vi "QAQC_vacoff.vi"() -> ()   [LabVIEW 2015]
uses:
  GlobalPath.vi
  GlobalData.vi
  GlobalVi.vi
panel:
  out "Mapping file Int sx":string
  out "Mapping file Int dx":string
  out "Mapping file Ext sx":string
  out "Mapping file Ext dx":string
  out "Mapping file pillar":string
  out "PanelName":string
  in  "DONE ALL?":bool
  in  "ptfe 6":bool caption="Open the vi for the QAQC planarity measurements of the frame+cooling bar region"
  in  "ptfe 3":bool caption="Remove the tooling from the table"
  in  "ptfe 5":bool caption="Open the vi for the QAQC planarity measurements of the pillar region"
  in  "ptfe 2":bool caption="Make sure the vacuum is switched OFF"
  # "1. QAQC with vacuum off"
  # "2. Start QAQC process"
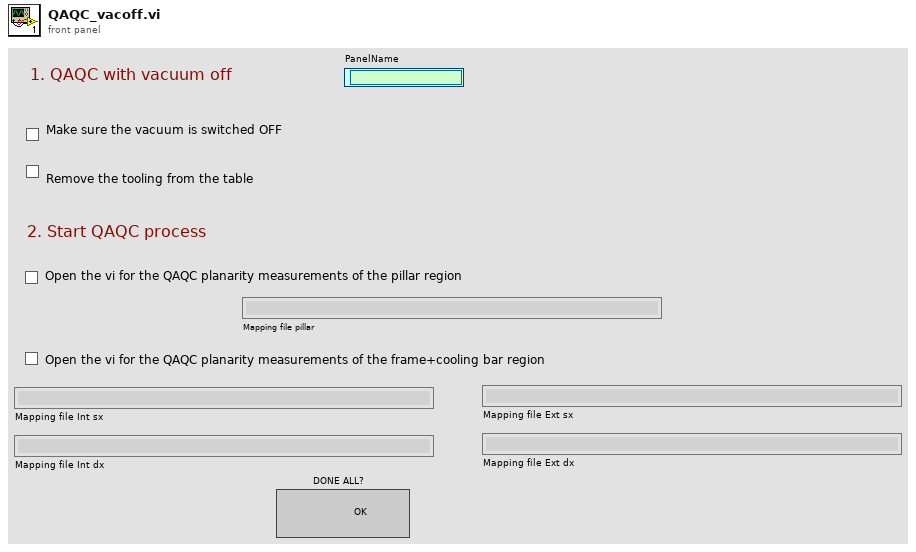
[diagram p1: front panel]
types:
  T1 = enum16{"open", "replace", "create", "open or create", "replace or create", "replace or create with confirmation"}
  T2 = enum32{"Bad", "Idle", "Run top level", "Running"}
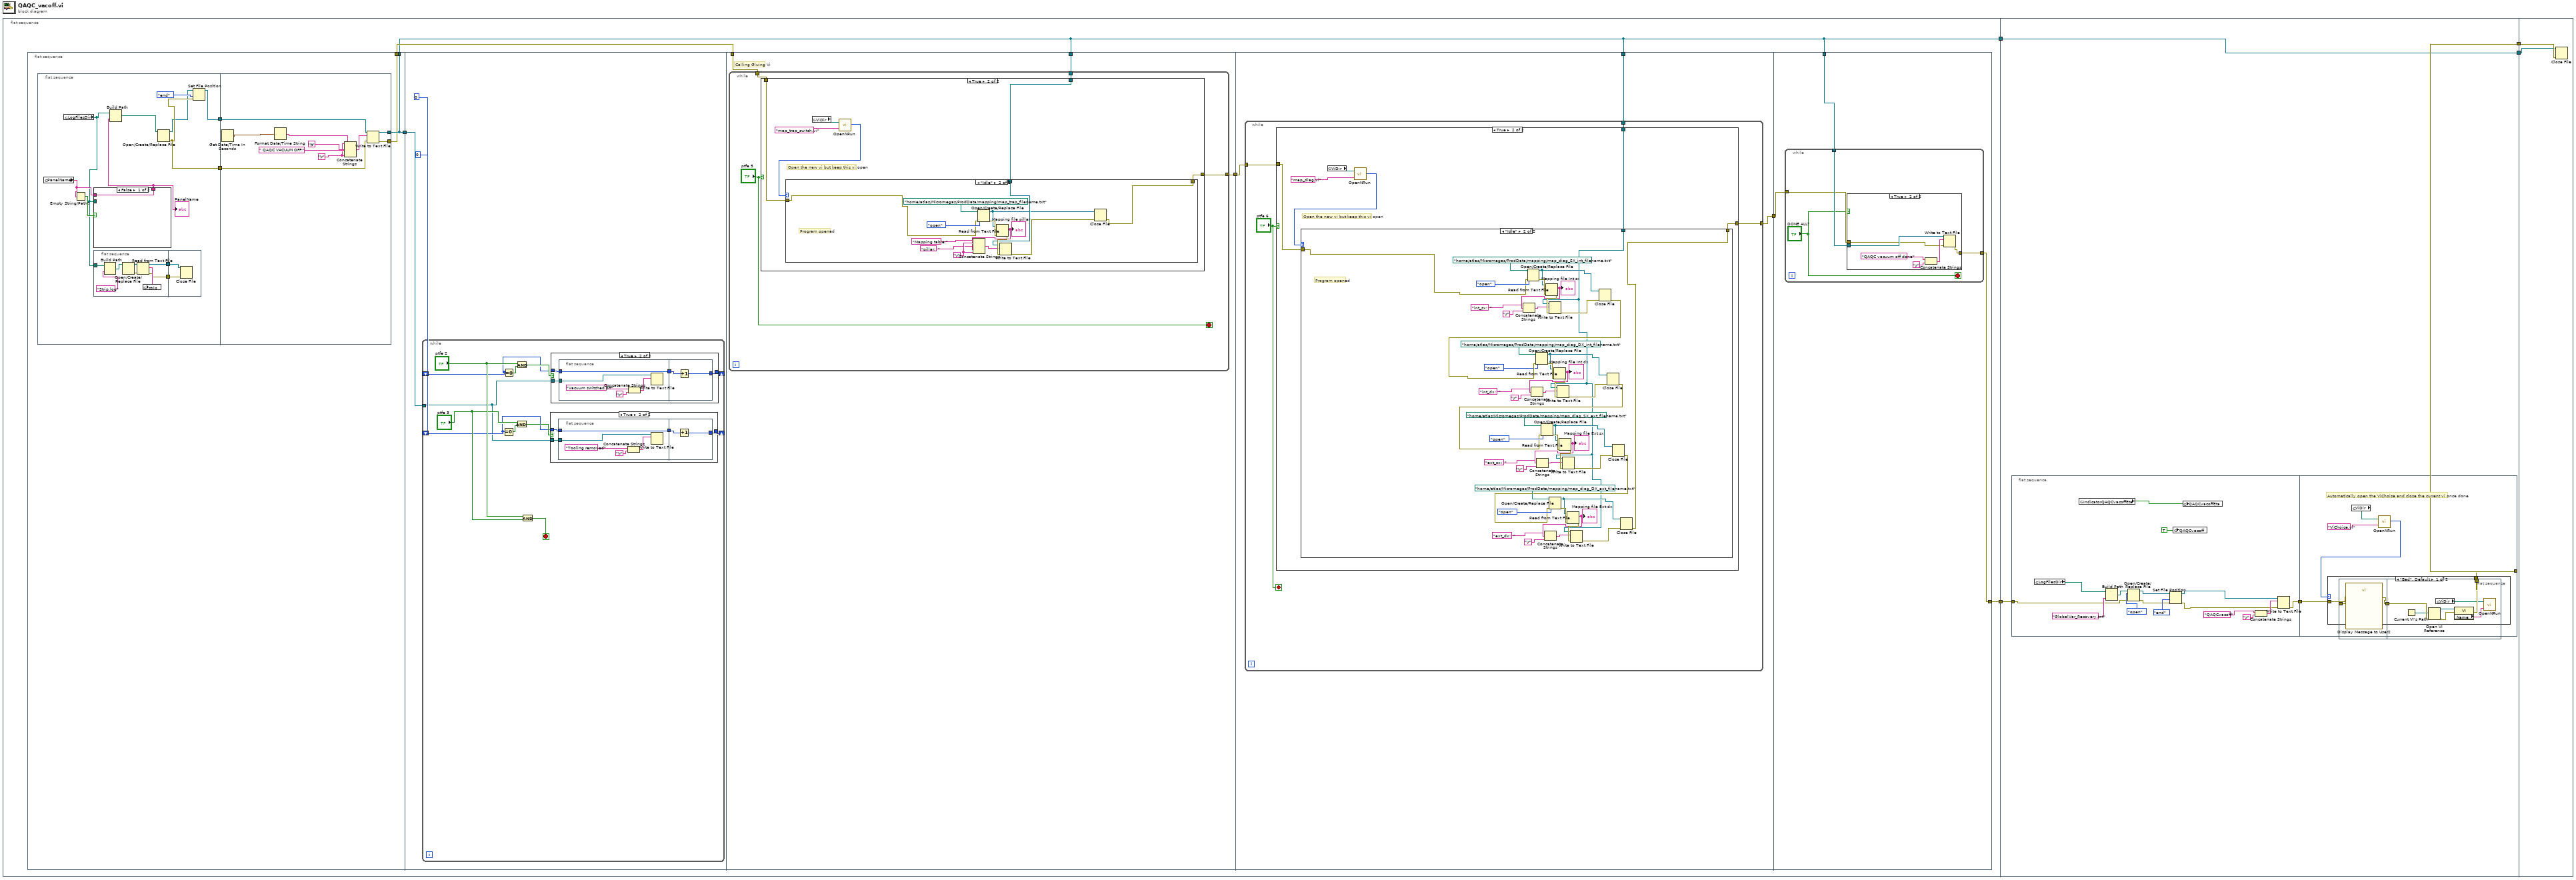
[diagram p0: block diagram]
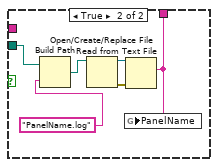
[diagram p2: hidden frame]
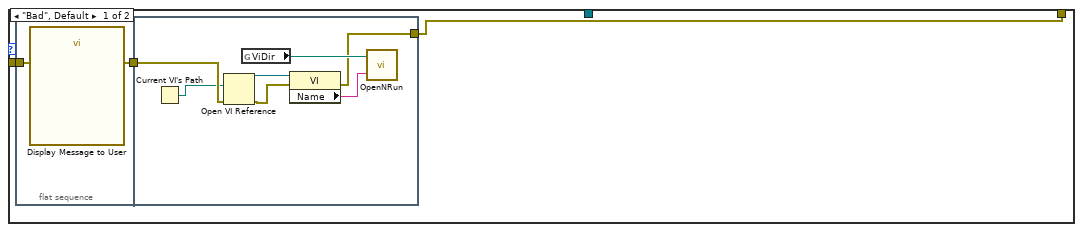
[diagram p6: hidden frame]
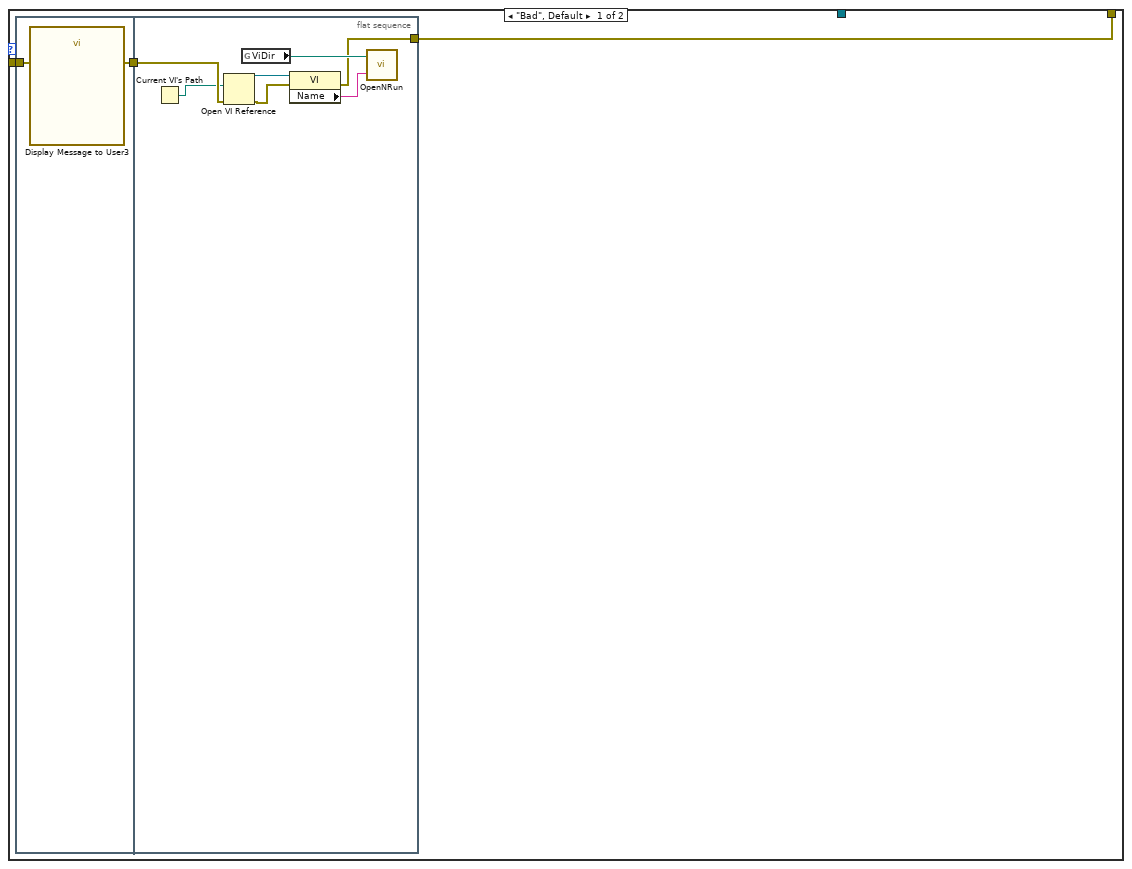
[diagram p8: hidden frame]
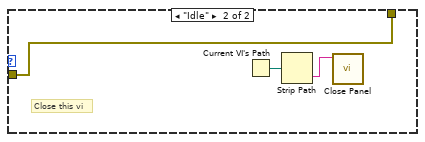
[diagram p10: hidden frame]
diagram:
  n1 = flat-sequence {
    tunnel: [w5] -> w3
    tunnel: [w6] -> w1
    tunnel: [w221] -> w4
    tunnel: w3 -> [w220]
    tunnel: [w220] -> w2
    tunnel: w1 -> [w218]
    tunnel: w4 -> [w259]
    tunnel: w2 -> [w258]
    frame #0 {
      n2 = flat-sequence {
        tunnel: [w13] -> w10
        tunnel: [w13] -> w5
        tunnel: [w12] -> w9
        tunnel: w10 -> [w55]
        tunnel: w9 -> [w94]
        tunnel: [w93] -> w8
        tunnel: w5 -> [w92]
        tunnel: w8 -> [w134]
        tunnel: [w133] -> w7
        tunnel: w5 -> [w132]
        tunnel: w5 -> [w206]
        tunnel: w7 -> [w205]
        tunnel: [w204] -> w6
        frame #0 {
          n3 = flat-sequence {
            tunnel: [w21] -> w14
            tunnel: [w23] -> w11
            tunnel: w14 -> [w48]
            tunnel: [w47] -> w13
            tunnel: [w46] -> w12
            tunnel: w11 -> [w45]
            frame #0 {
              n4 = global read "GlobalData.vi" "PanelName"() -> (w19:string)
              n5 = global read "GlobalPath.vi" "LogFilesDir"() -> (w15:path)
              n6 = Empty String/Path?(string/path=w19) -> (empty?=w20:bool)
              n7 = case shown="False" w20 {
                tunnel: w15 -> [_ w42]
                tunnel: [w36 w37] -> w18
                tunnel: w19 -> [w36 _]
                frame False {
                }
                frame True {
                  n8 = Build Path(base path=w42, name or relative path="PanelName.log") -> (appended path=w41:path)
                  n9 = Open/Create/Replace File(file path (use dialog)=w41) -> (refnum out=w38:refnum<file>, error out=w39:errorcluster)  [unwired: 5 in, 1 out]
                  n10 = Read from Text File(file (use dialog)=w38, error in=w39) -> (text=w37:string)  [unwired: 2 in, 3 out]
                  n11 = global write "GlobalData.vi" "PanelName"(w37) -> ()
                }
              }
              "PanelName" <- w18
              n12 = flat-sequence {
                tunnel: w15 -> [w33]
                tunnel: [w27] -> w17
                tunnel: [w26] -> w16
                tunnel: w17 -> [w35]
                tunnel: w16 -> [w34]
                frame #0 {
                  n13 = Build Path(base path=w33, name or relative path="Strip.log") -> (appended path=w32:path)
                  n14 = Open/Create/Replace File(file path (use dialog)=w32) -> (refnum out=w29:refnum<file>, error out=w30:errorcluster)  [unwired: 5 in, 1 out]
                  n15 = Read from Text File(file (use dialog)=w29, error in=w30) -> (refnum out=w26:refnum<file>, text=w28:string, error out=w27:errorcluster)  [unwired: 2 in, 1 out]
                  n16 = global write "GlobalData.vi" "strip"(w28) -> ()
                }
                frame #1 {
                  n17 = Close File(refnum=w34, error in=w35) -> ()  [unwired: 2 out]
                }
              }
              n18 = Build Path(base path=w15, name or relative path=w18) -> (appended path=w25:path)
              n19 = Open/Create/Replace File(file path (use dialog)=w25) -> (refnum out=w22:refnum<file>, error out=w23:errorcluster)  [unwired: 5 in, 1 out]
              n20 = Set File Position(refnum=w22, from (0:start)=enum16{"start", "end", "current"}."end", error in=w23) -> (refnum out=w21:refnum<file>)  [unwired: 1 in, 1 out]
            }
            frame #1 {
              w43 = "\r"
              n21 = Get Date/Time In Seconds() -> (seconds since 1Jan1904=w44:timestamp)
              n22 = Format Date/Time String(seconds (now)=w44) -> (date/time string=w50:string)  [unwired: 2 in]
              n23 = Concatenate Strings(w43, w50, "\t", " QAQC VACUUM OFF:", w43) -> (w49:string)
              n24 = Write to Text File(file (use dialog)=w48, text=w49, error in=w45) -> (refnum out=w47:refnum<file>, error out=w46:errorcluster)  [unwired: 1 in, 1 out]
            }
          }
        }
        frame #1 {
          n25 = while {
            tunnel: w55 -> [w56]
            shift-right: [w62] -> _
            shift-left: 0 -> [w63]
            shift-right: [w57] -> _
            shift-left: 0 -> [w58]
            stop <- w67 stop-if-true
            n26 = Equal To 0?(x=w58) -> (x = 0?=w61:bool)
            n27 = Equal To 0?(x=w63) -> (x = 0?=w66:bool)
            n28 = And(x="ptfe 3", y=w61) -> (x .and. y?=w60:bool)
            n29 = And(x="ptfe 2", y=w66) -> (x .and. y?=w65:bool)
            n30 = Compound Arithmetic op=AND("ptfe 2", "ptfe 3") -> (w67:bool)
            n31 = case shown="True" w60 {
              tunnel: w56 -> [_ w72]
              tunnel: w58 -> [w68 w70]
              tunnel: [w68 w69] -> w57
              frame False {
              }
              frame True {
                n32 = flat-sequence {
                  tunnel: w72 -> [w75]
                  tunnel: [w74] -> w71
                  tunnel: w70 -> [w74]
                  tunnel: w71 -> [w79]
                  tunnel: [w78] -> w69
                  frame #0 {
                    n33 = Concatenate Strings("Tooling removed", "\r") -> (w77:string)
                    n34 = Write to Text File(file (use dialog)=w75, text=w77) -> ()  [unwired: 2 in, 3 out]
                  }
                  frame #1 {
                    n35 = Increment(x=w79) -> (x+1=w78:i32)
                  }
                }
              }
            }
            n36 = case shown="True" w65 {
              tunnel: w56 -> [_ w84]
              tunnel: w63 -> [w80 w82]
              tunnel: [w80 w81] -> w62
              frame False {
              }
              frame True {
                n37 = flat-sequence {
                  tunnel: w84 -> [w87]
                  tunnel: [w86] -> w83
                  tunnel: w82 -> [w86]
                  tunnel: w83 -> [w91]
                  tunnel: [w90] -> w81
                  frame #0 {
                    n38 = Concatenate Strings("Vacuum switched off", "\r") -> (w89:string)
                    n39 = Write to Text File(file (use dialog)=w87, text=w89) -> ()  [unwired: 2 in, 3 out]
                  }
                  frame #1 {
                    n40 = Increment(x=w91) -> (x+1=w90:i32)
                  }
                }
              }
            }
          }
        }
        frame #2 {
          # "Calling Gluing Vi"
          n41 = while {
            tunnel: w94 -> [w98]
            tunnel: [w97] -> w93
            tunnel: w92 -> [w95]
            stop <- "ptfe 5" stop-if-true
            n42 = case shown="True" "ptfe 5" {
              tunnel: w98 -> [w99 w102]
              tunnel: [w99 w101] -> w97
              tunnel: w95 -> [_ w100]
              frame False {
              }
              frame True {
                # "Open the new vi but keep this vi open"
                n43 = global read "GlobalPath.vi" "ViDir"() -> (w105:path)
                n44 = call "OpenNRun.vi"("VI name"="map_trap_switch.vi", "ViDirPath"=w105) -> ("Execution:State"=w104:T2)
                n45 = case shown="\"Idle\"" w104 {
                  tunnel: [w106 w120] -> w101
                  tunnel: w102 -> [w108 w121]
                  tunnel: w100 -> [_ w122]
                  frame "Bad", Default {
                    n46 = flat-sequence {
                      tunnel: w108 -> [w109]
                      tunnel: [w110] -> w107
                      tunnel: w107 -> [w114]
                      tunnel: [w111] -> w106
                      frame #0 {
                        n47 = call "Display Message to User"("error in (no error)"=w109) -> ("error out"=w110:errorcluster)  [unwired: 9 in, 1 out]
                      }
                      frame #1 {
                        n48 = Current VI's Path() -> (path=w112:path)
                        n49 = Open VI Reference(vi path=w112, error in (no error)=w114) -> (vi reference=w117:refnum<vi>, error out=w116:errorcluster)  [unwired: 4 in]
                        n50 = global read "GlobalPath.vi" "ViDir"() -> (w113:path)
                        n51 = property class="VI"(reference=w117, error in=w116) -> (error out=w111:errorcluster, "Name"=w115:string)  [unwired: 1 out]
                        n52 = call "OpenNRun.vi"("VI name"=w115, "ViDirPath"=w113) -> ()  [unwired: 1 out]
                      }
                    }
                  }
                  frame "Idle" {
                    w125 = "\r"
                    # "Program opened"
                    n53 = Open/Create/Replace File(file path (use dialog)=path "/home/atlas/Micromegas/ProdData/mapping/map_trap_filename.txt", error in=w121, operation (0:open)=T1."open") -> (refnum out=w118:refnum<file>, error out=w129:errorcluster)  [unwired: 3 in, 1 out]
                    n54 = Read from Text File(file (use dialog)=w118, error in=w129) -> (text=w124:string, error out=w128:errorcluster)  [unwired: 2 in, 2 out]
                    "Mapping file pillar" <- w124
                    n55 = Concatenate Strings("Mapping table:", w125, "pillar:  ", w124, w125) -> (w127:string)
                    n56 = Write to Text File(file (use dialog)=w122, text=w127, error in=w128) -> (error out=w119:errorcluster)  [unwired: 1 in, 2 out]
                    n57 = Close File(refnum=w118, error in=w119) -> (error out=w120:errorcluster)  [unwired: 1 out]
                  }
                }
              }
            }
          }
        }
        frame #3 {
          n58 = while {
            tunnel: [w138] -> w133
            tunnel: w134 -> [w136]
            tunnel: w132 -> [w135]
            stop <- "ptfe 6" stop-if-true
            n59 = case shown="True" "ptfe 6" {
              tunnel: w136 -> [w139 w142]
              tunnel: [w139 w141] -> w138
              tunnel: w135 -> [_ w140]
              frame False {
              }
              frame True {
                # "Open the new vi but keep this vi open"
                n60 = global read "GlobalPath.vi" "ViDir"() -> (w145:path)
                n61 = call "OpenNRun.vi"("VI name"="map_diag.vi", "ViDirPath"=w145) -> ("Execution:State"=w144:T2)
                n62 = case shown="\"Idle\"" w144 {
                  tunnel: [w146 w160] -> w141
                  tunnel: w142 -> [w148 w158]
                  tunnel: w140 -> [_ w159]
                  frame "Bad", Default {
                    n63 = flat-sequence {
                      tunnel: w148 -> [w149]
                      tunnel: [w150] -> w147
                      tunnel: w147 -> [w154]
                      tunnel: [w151] -> w146
                      frame #0 {
                        n64 = call "Display Message to User3"("error in (no error)"=w149) -> ("error out"=w150:errorcluster)  [unwired: 9 in, 1 out]
                      }
                      frame #1 {
                        n65 = Current VI's Path() -> (path=w152:path)
                        n66 = Open VI Reference(vi path=w152, error in (no error)=w154) -> (vi reference=w157:refnum<vi>, error out=w156:errorcluster)  [unwired: 4 in]
                        n67 = global read "GlobalPath.vi" "ViDir"() -> (w153:path)
                        n68 = property class="VI"(reference=w157, error in=w156) -> (error out=w151:errorcluster, "Name"=w155:string)  [unwired: 1 out]
                        n69 = call "OpenNRun.vi"("VI name"=w155, "ViDirPath"=w153) -> ()  [unwired: 1 out]
                      }
                    }
                  }
                  frame "Idle" {
                    # "Program opened"
                    n70 = Open/Create/Replace File(file path (use dialog)=path "/home/atlas/Micromegas/ProdData/mapping/map_diag_SX_int_filename.txt", error in=w158, operation (0:open)=T1."open") -> (refnum out=w193:refnum<file>, error out=w200:errorcluster)  [unwired: 3 in, 1 out]
                    n71 = Read from Text File(file (use dialog)=w193, error in=w200) -> (text=w196:string, error out=w199:errorcluster)  [unwired: 2 in, 2 out]
                    "Mapping file Int sx" <- w196
                    n72 = Concatenate Strings("int_sx:  ", w196, "\r") -> (w198:string)
                    n73 = Write to Text File(file (use dialog)=w159, text=w198, error in=w199) -> (error out=w194:errorcluster)  [unwired: 1 in, 2 out]
                    n74 = Close File(refnum=w193, error in=w194) -> (error out=w203:errorcluster)  [unwired: 1 out]
                    n75 = Open/Create/Replace File(file path (use dialog)=path "/home/atlas/Micromegas/ProdData/mapping/map_diag_DX_int_filename.txt", error in=w203, operation (0:open)=T1."open") -> (refnum out=w183:refnum<file>, error out=w190:errorcluster)  [unwired: 3 in, 1 out]
                    n76 = Read from Text File(file (use dialog)=w183, error in=w190) -> (text=w186:string, error out=w189:errorcluster)  [unwired: 2 in, 2 out]
                    "Mapping file Int dx" <- w186
                    n77 = Concatenate Strings("int_dx:  ", w186, "\r") -> (w188:string)
                    n78 = Write to Text File(file (use dialog)=w159, text=w188, error in=w189) -> (error out=w184:errorcluster)  [unwired: 1 in, 2 out]
                    n79 = Close File(refnum=w183, error in=w184) -> (error out=w172:errorcluster)  [unwired: 1 out]
                    n80 = Open/Create/Replace File(file path (use dialog)=path "/home/atlas/Micromegas/ProdData/mapping/map_diag_SX_ext_filename.txt", error in=w172, operation (0:open)=T1."open") -> (refnum out=w173:refnum<file>, error out=w180:errorcluster)  [unwired: 3 in, 1 out]
                    n81 = Read from Text File(file (use dialog)=w173, error in=w180) -> (text=w176:string, error out=w179:errorcluster)  [unwired: 2 in, 2 out]
                    "Mapping file Ext sx" <- w176
                    n82 = Concatenate Strings("ext_sx:  ", w176, "\r") -> (w178:string)
                    n83 = Write to Text File(file (use dialog)=w159, text=w178, error in=w179) -> (error out=w174:errorcluster)  [unwired: 1 in, 2 out]
                    n84 = Close File(refnum=w173, error in=w174) -> (error out=w161:errorcluster)  [unwired: 1 out]
                    n85 = Open/Create/Replace File(file path (use dialog)=path "/home/atlas/Micromegas/ProdData/mapping/map_diag_DX_ext_filename.txt", error in=w161, operation (0:open)=T1."open") -> (refnum out=w162:refnum<file>, error out=w169:errorcluster)  [unwired: 3 in, 1 out]
                    n86 = Read from Text File(file (use dialog)=w162, error in=w169) -> (text=w165:string, error out=w168:errorcluster)  [unwired: 2 in, 2 out]
                    "Mapping file Ext dx" <- w165
                    n87 = Concatenate Strings("ext_dx:  ", w165, "\r") -> (w167:string)
                    n88 = Write to Text File(file (use dialog)=w159, text=w167, error in=w168) -> (error out=w163:errorcluster)  [unwired: 1 in, 2 out]
                    n89 = Close File(refnum=w162, error in=w163) -> (error out=w160:errorcluster)  [unwired: 1 out]
                  }
                }
              }
            }
          }
        }
        frame #4 {
          n90 = while {
            tunnel: w206 -> [w210]
            tunnel: w205 -> [w209]
            tunnel: [w207] -> w204
            stop <- "DONE ALL?" stop-if-true
            n91 = case shown="True" "DONE ALL?" {
              tunnel: w210 -> [_ w214]
              tunnel: w209 -> [w211 w213]
              tunnel: [w211 w212] -> w207
              frame False {
              }
              frame True {
                n92 = Concatenate Strings("QAQC vacuum off done", "\r") -> (w217:string)
                n93 = Write to Text File(file (use dialog)=w214, text=w217, error in=w213) -> (error out=w212:errorcluster)  [unwired: 1 in, 2 out]
              }
            }
          }
        }
      }
    }
    frame #1 {
      n94 = flat-sequence {
        tunnel: w218 -> [w225]
        tunnel: [w226] -> w219
        tunnel: [w239] -> w221
        tunnel: w219 -> [w238]
        frame #0 {
          n95 = global read "GlobalPath.vi" "LogFilesDir"() -> (w223:path)
          n96 = global read "GlobalVi.vi" "IndicatorQAQCvacoffEta"() -> (w222:bool)
          n97 = Build Path(base path=w223, name or relative path="GlobalVar_Recovery.txt") -> (appended path=w235:path)
          n98 = Open/Create/Replace File(file path (use dialog)=w235, error in=w225, operation (0:open)=T1."open") -> (refnum out=w231:refnum<file>, error out=w232:errorcluster)  [unwired: 3 in, 1 out]
          n99 = Set File Position(refnum=w231, from (0:start)=enum16{"start", "end", "current"}."end", error in=w232) -> (refnum out=w228:refnum<file>, error out=w227:errorcluster)  [unwired: 1 in]
          n100 = global write "GlobalVi.vi" "QAQCvacoff"(TRUE) -> ()
          n101 = global write "GlobalVi.vi" "QAQCvacoffEta"(w222) -> ()
          n102 = Concatenate Strings("QAQCvacoff", "\r") -> (w230:string)
          n103 = Write to Text File(file (use dialog)=w228, text=w230, error in=w227) -> (error out=w226:errorcluster)  [unwired: 1 in, 2 out]
        }
        frame #1 {
          # "Automatically open the ViChoise and close the current vi once done"
          n104 = global read "GlobalPath.vi" "ViDir"() -> (w242:path)
          n105 = call "OpenNRun.vi"("VI name"="ViChoice.vi", "ViDirPath"=w242) -> ("Execution:State"=w241:T2)
          n106 = case shown="\"Bad\", Default" w241 {
            tunnel: [w245 w257] -> w239
            tunnel: w238 -> [w244 w257]
            frame "Bad", Default {
              n107 = flat-sequence {
                tunnel: w244 -> [w247]
                tunnel: [w246] -> w243
                tunnel: [w251] -> w245
                tunnel: w243 -> [w250]
                frame #0 {
                  n108 = call "Display Message to User2"("error in (no error)"=w247) -> ("error out"=w246:errorcluster)  [unwired: 9 in, 1 out]
                }
                frame #1 {
                  n109 = Current VI's Path() -> (path=w248:path)
                  n110 = Open VI Reference(vi path=w248, error in (no error)=w250) -> (vi reference=w254:refnum<vi>, error out=w253:errorcluster)  [unwired: 4 in]
                  n111 = global read "GlobalPath.vi" "ViDir"() -> (w249:path)
                  n112 = property class="VI"(reference=w254, error in=w253) -> (error out=w251:errorcluster, "Name"=w252:string)  [unwired: 1 out]
                  n113 = call "OpenNRun.vi"("VI name"=w252, "ViDirPath"=w249) -> ()  [unwired: 1 out]
                }
              }
            }
            frame "Idle" {
              # "Close this vi"
              n114 = Current VI's Path() -> (path=w256:path)
              n115 = Strip Path(path=w256) -> (name=w255:string)  [unwired: 1 out]
              n116 = call <vilib>:"Close Panel.vi"("VI name"=w255) -> ()  [unwired: 10 in, 1 out]
            }
          }
        }
      }
    }
    frame #2 {
      n117 = Close File(refnum=w258, error in=w259) -> ()  [unwired: 2 out]
    }
  }
